vi "Read Class Path.vi"(8 "error in (no error)":errorcluster, 11 "Usuarios in":refnum<class "Usuarios.lvclass">) -> (0 "error out":errorcluster, 2 "Class Path":path, 3 "Usuarios out":refnum<class "Usuarios.lvclass">)   [LabVIEW 2019, in "Usuarios.lvclass"]
uses:
  Usuarios.lvclass
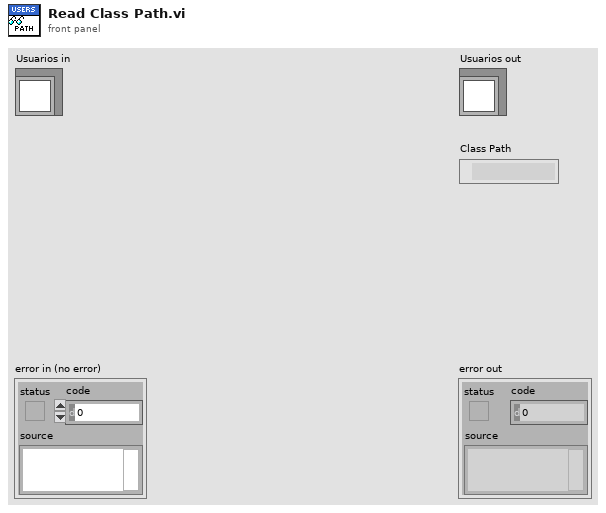
[diagram p1: front panel]
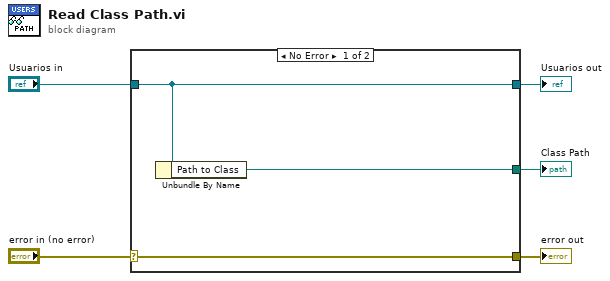
[diagram p0: block diagram]
diagram:
  n1 = case shown="No Error" "error in (no error)" {
    selector: "error in (no error)" -> [w8 w9]
    tunnel: [w8 w9] -> w4
    tunnel: [w7 w10] -> w2
    tunnel: "Usuarios in" -> [w7 w10]
    tunnel: [w6 _] -> w1
    frame No Error {
      n2 = Unbundle By Name(w7) -> ("Path to Class"=w6:path)
    }
    frame Error {
    }
  }
  "error out" <- w4
  "Usuarios out" <- w2
  "Class Path" <- w1
